vi "setREF_TC.vi"(8 "error in (no error)":errorcluster, 9 "TC (s)":dbl=1e-05 min=0.0001 format="%#_3p", 10 "REF Channel":i32=1 min=1 max=16, 11 "Instrument.LockinAPI in":refnum<class "Instrument.LockinAPI.lvclass">) -> (0 "error out":errorcluster, 3 "Instrument.LockinAPI out":refnum<class "Instrument.LockinAPI.lvclass">)   [LabVIEW 2019, in "Instrument.LockinAPI.lvclass"]
doc: "API to configure a REF frequency.\n\nSpecify which channel you want to change and the value you want to set.\n\nIf address=\"\", this API reads from localhost\nIf address is remote lockin, you need to add this computer to allowed whitelist on the lockin computer you are trying to access."
uses:
  Instrument.LockinAPI.lvclass
  C:/Users/patrick/Documents/GitHub/Instrument-Framework/lvsrc/Instrument/Instrument.lvclass
  Typedefs/LockinAPI.Commands--Enum.ctl
  Typedefs/LockinAPI.setREF_TC--cluster.ctl
  85235deb-aab8-4569-a361-c3224e699e15.vi
  85235deb-aab8-4569-a361-c3224e699e15.vi/15fb9db0-95b5-4893-9bd7-ff8e2cca8b77.vi
  85235deb-aab8-4569-a361-c3224e699e15.vi/15fb9db0-95b5-4893-9bd7-ff8e2cca8b77.vi/d2602330-76c0-4da6-bc07-f421da57d6a6.vi
  85235deb-aab8-4569-a361-c3224e699e15.vi/15fb9db0-95b5-4893-9bd7-ff8e2cca8b77.vi/025d6ff1-ffb0-406f-bd3b-4e34afee9e72.vi
  Instrument/Protected/Validate API method.vi
  Instrument/Private/Get RC Connection Status.vi
  Instrument/API/Send and Receive.vi
  <vilib>/Utility/Data Type/Get Type Information.vi
  <vilib>/JDP Science/JSONtext/JSON text to Variant.vi
  <vilib>/JDP Science/JSONtext/LVClass Serializer/JSONtext LVClass Serializer.lvclass
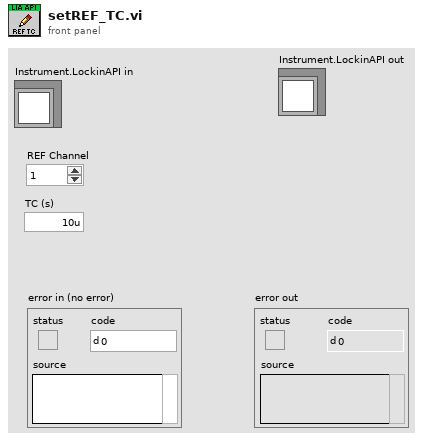
[diagram p1: front panel]
types:
  T1 = typedef "Instrument.LockinAPI.lvclass/LockinAPI.setREF_TC--cluster.ctl" = cluster{"REF Channel":i32, "TC (s)":dbl}
  T2 = typedef "Instrument.LockinAPI.lvclass/LockinAPI.Commands--Enum.ctl" = enum16{"setAI", "setAO", "setAO_Amplitude", "setAO_DC", "setAO_Frequency", "setAO_Phase", "setAO_Function", "setAO_I+", "setREF", "setREF_Frequency", "setREF_Phase", "setREF_TC", "setREF_Roll-Off", "setDAQ", "setSampling", "setOffset", "setState", "getState", "getAO", "getAI", "getResults", "getSampling", "getAOconfig", "getREFconfig", "setInputGain", "setOutputGain", "getInputGain", "getOutputGain", "setSamplingMode", "getSamplingMode", "setSweep", "setSweepTime", "setSweepTable", "getStatus", "getSweepResults", "getSweepWaveforms", "startSweep", "stopSweep", "setAUX", "getAUX"}
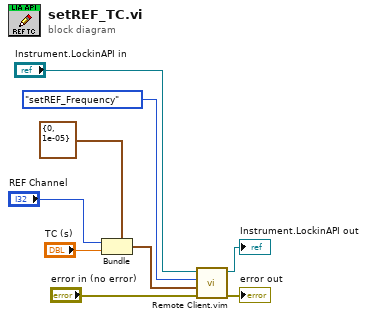
[diagram p0: block diagram]
diagram:
  n1 = Bundle(cluster=T1 {"REF Channel"=0, "TC (s)"=1e-05} ("setREF_phi"), "REF Channel"="REF Channel", "TC (s)"="TC (s)") -> (w4:T1)
  n2 = call "Remote Client.vim"("error in (no error)"="error in (no error)", "Data in"=w4, "Command in"=LockinAPI.Commands--Enum."setREF_Frequency" ("Command"), "Instrument in"="Instrument.LockinAPI in") -> ("error out"=→"error out":errorcluster, "Instrument out"=→"Instrument.LockinAPI out":refnum<class "Instrument.LockinAPI.lvclass">)  [unwired: 4 in, 2 out]
